vi "GetSourceAndSinkTerminals.vi"(8 "error in (no error)":errorcluster, 11 "Terms[]":refnum<vi>[](array[refnum])) -> (0 "error out":errorcluster, 2 "Sink":refnum<vi>[](array[refnum]), 3 "Source":refnum<vi>[](array[refnum]))   [LabVIEW 2014]
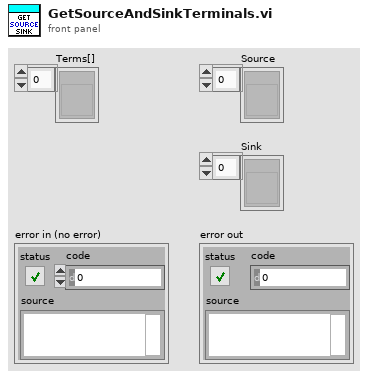
[diagram p1: front panel]
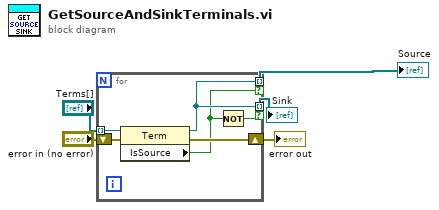
[diagram p0: block diagram]
diagram:
  n1 = for {
    tunnel: "Terms[]" -> [w9] mode=indexing
    shift-right: [w10] -> w4
    shift-left: "error in (no error)" -> [w11]
    tunnel: [w8] -> w5 mode=indexing if=w7
    tunnel: [w8] -> w3 mode=indexing if=w6
    n2 = property class="Term"(reference=w9, error in=w11) -> (reference out=w8:refnum<vi>, error out=w10:errorcluster, "IsSource"=w7:bool)
    n3 = Not(x=w7) -> (.not. x?=w6:bool)
  }
  "Source" <- w5
  "error out" <- w4
  "Sink" <- w3
